vi "Show Sequence.vi"(8 "error in (no error)":errorcluster, 10 "Sequence":string, 11 "SequenceViewPanel in":refnum<class "SequenceViewPanel.lvclass">) -> (0 "error out":errorcluster, 3 "SequenceViewPanel out":refnum<class "SequenceViewPanel.lvclass">)   [LabVIEW 2020, in "TSnax UI.lvlib" / "SequenceViewPanel.lvclass"]
uses:
  SequenceViewPanel.lvclass
  TSnax/Sequence/Step Group.ctl
  SequenceViewPanel.lvclass/SequenceViewPanel.ctl
  TSnax/SequenceFile/SequenceFile.lvclass
  TSnax/Sequence/Sequence.lvclass
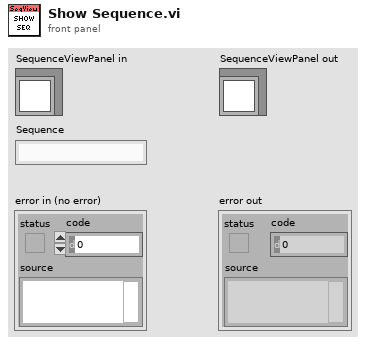
[diagram p1: front panel]
types:
  T1 = typedef "TSnax.lvlib/Sequence.lvclass/Step Group.ctl" = enum16{"Setup", "Main", "Cleanup"}
  T2 = typedef "TSnax UI.lvlib/SequenceViewPanel.lvclass/Ref Data.ctl" = cluster{"Insert Index":i32, "SequenceFile":refnum<class "SequenceFile.lvclass">, "Sequence":string}
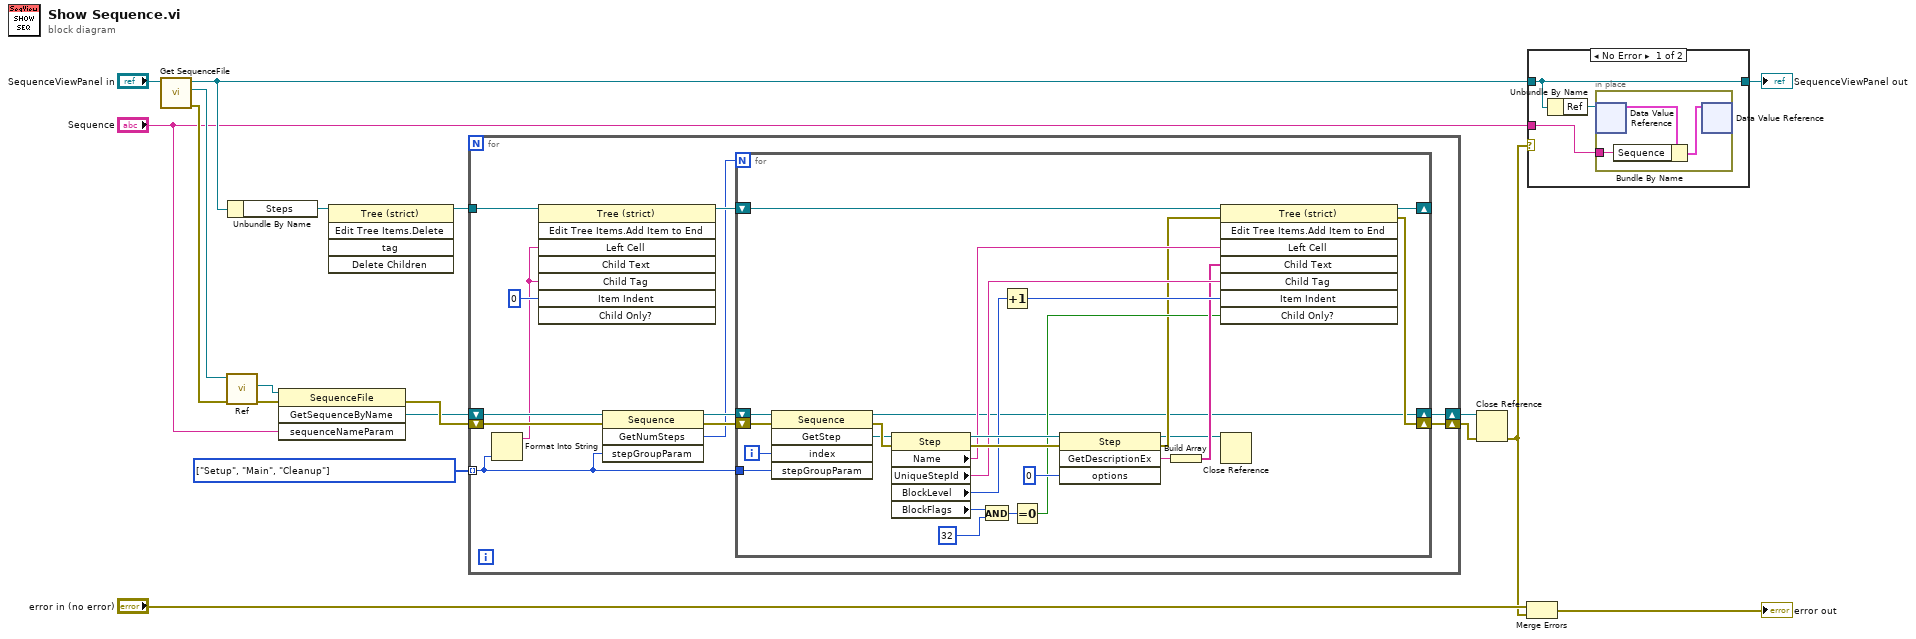
[diagram p0: block diagram]
diagram:
  w10 = T1[] [enum."Setup", enum."Main", enum."Cleanup"] items=["Setup", "Main", "Cleanup"]
  n1 = call "Get SequenceFile.vi"("SequenceViewPanel in"="SequenceViewPanel in") -> ("error out"=w14:errorcluster, "SequenceFile"=w15:refnum<class "SequenceFile.lvclass">, "SequenceViewPanel out"=w4:refnum<class "SequenceViewPanel.lvclass">)  [unwired: 8 in]
  n2 = call "Ref.vi"("error in (no error)"=w14, "SequenceFile in"=w15) -> ("error out"=w12:errorcluster, "Ref"=w13:refnum<k7>)  [unwired: 7 in, 1 out]
  n3 = Unbundle By Name(w4) -> ("Steps"=w9:refnum<vi>)
  n4 = invoke class="SequenceFile" method="GetSequenceByName"(reference=w13, error in=w12, "sequenceNameParam"="Sequence") -> (error out=w18:errorcluster, "GetSequenceByName"=w11:refnum<k7>)  [unwired: 1 in, 2 out]
  n5 = invoke class="Tree (strict)" method="Edit Tree Items.Delete"(reference=w9) -> (reference out=w8:refnum<vi>)  [unwired: 4 in, 4 out]
  n6 = for {
    tunnel: w10 -> [w21] mode=indexing
    tunnel: w8 -> [w28]
    shift-right: [w19] -> w6
    shift-left: w18 -> [w30]
    shift-right: [w20] -> w7
    shift-left: w11 -> [w29]
    n7 = Format Into String(w21) -> (resulting string=w26:string)  [unwired: 3 in, 1 out]
    n8 = invoke class="Tree (strict)" method="Edit Tree Items.Add Item to End"(reference=w28, "Left Cell"=w26, "Child Tag"=w26, "Item Indent"=0 ("New Item Indentation")) -> (reference out=w25:refnum<vi>)  [unwired: 4 in, 7 out]
    n9 = invoke class="Sequence" method="GetNumSteps"(reference=w29, error in=w30, "stepGroupParam"=w21) -> (reference out=w24:refnum<k7>, error out=w23:errorcluster, "GetNumSteps"=w22:i32)  [unwired: 1 in, 1 out]
    n10 = for {
      N: w22 -> [_]
      shift-right: [w34] -> _
      shift-left: w25 -> [w36]
      shift-right: [w31] -> w20
      shift-left: w24 -> [w54]
      shift-right: [w33] -> w19
      shift-left: w23 -> [w53]
      tunnel: w21 -> [w51]
      i -> [w52]
      n11 = invoke class="Sequence" method="GetStep"(reference=w54, error in=w53, "index"=w52, "stepGroupParam"=w51) -> (reference out=w31:refnum<k7>, error out=w55:errorcluster, "GetStep"=w50:refnum<k7>)  [unwired: 1 in, 2 out]
      n12 = property class="Step"(reference=w50, error in=w55) -> (reference out=w49:refnum<k7>, error out=w48:errorcluster, "Name"=w46:string, "UniqueStepId"=w45:string, "BlockLevel"=w44:i32, "BlockFlags"=w42:i32)
      n13 = And(x=w42, y=32) -> (x .and. y?=w38:i32)
      n14 = Increment(x=w44) -> (x+1=w43:i32)
      n15 = Equal To 0?(x=w38) -> (x = 0?=w37:bool)
      n16 = invoke class="Step" method="GetDescriptionEx"(reference=w49, error in=w48, "options"=0) -> (reference out=w32:refnum<k7>, error out=w35:errorcluster, "GetDescriptionEx"=w40:string)  [unwired: 1 in, 1 out]
      n17 = Build Array(w40) -> (w39:string[])
      n18 = invoke class="Tree (strict)" method="Edit Tree Items.Add Item to End"(reference=w36, error in=w35, "Left Cell"=w46, "Child Text"=w39, "Child Tag"=w45, "Item Indent"=w43, "Child Only?"=w37) -> (reference out=w34:refnum<vi>, error out=w33:errorcluster)  [unwired: 1 in, 6 out]
      n19 = Close Reference(reference=w32) -> ()  [unwired: 1 in, 1 out]
    }
  }
  n20 = Close Reference(reference=w7, error in (no error)=w6) -> (error out=w3:errorcluster)
  n21 = Merge Errors("error in (no error)", w3) -> (→"error out":errorcluster)
  n22 = case shown="No Error" w3 {
    tunnel: w4 -> [w57 w62]
    tunnel: [w57 w62] -> w2
    tunnel: "Sequence" -> [w56 _]
    frame No Error {
      n23 = Unbundle By Name(w57) -> ("Ref"=w58:refnum<data-value>)
      n24 = in-place {
        in-place-border: w56 -> [w59]
        n25 = in-place-dvr #1(w58) -> (w61:T2)  [unwired: 1 out]
        n26 = Bundle By Name(cluster=w61, "Sequence"=w59) -> (w60:T2)
        n27 = in-place-dvr #1(w60) -> ()  [unwired: 2 out]
      }
    }
    frame Error {
    }
  }
  "SequenceViewPanel out" <- w2
